vi "sort_points_iterative_closest_point.vi"(2 "Detected Camera Coordinates":cluster{"X":dbl, "Y":dbl}[](array[cluster]), 3 "Anticipated Camera Coordinates":cluster{"X":dbl, "Y":dbl}[](array[cluster]), 4 "Corresponding Projector Coordinates":cluster{"X":dbl, "Y":dbl}[](array[cluster])) -> (0 "Detected Camera Coordinates Sorted":cluster{"X":dbl, "Y":dbl}[](array[cluster]), 1 "Corresponding Projector Coordinates Filtered":cluster{"X":dbl, "Y":dbl}[](array[cluster]))   [LabVIEW 2019]
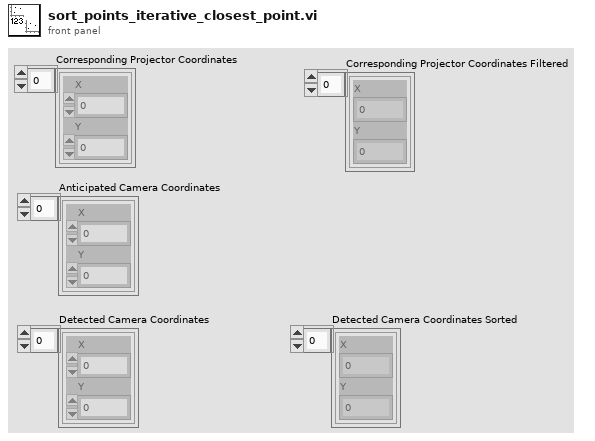
[diagram p1: front panel]
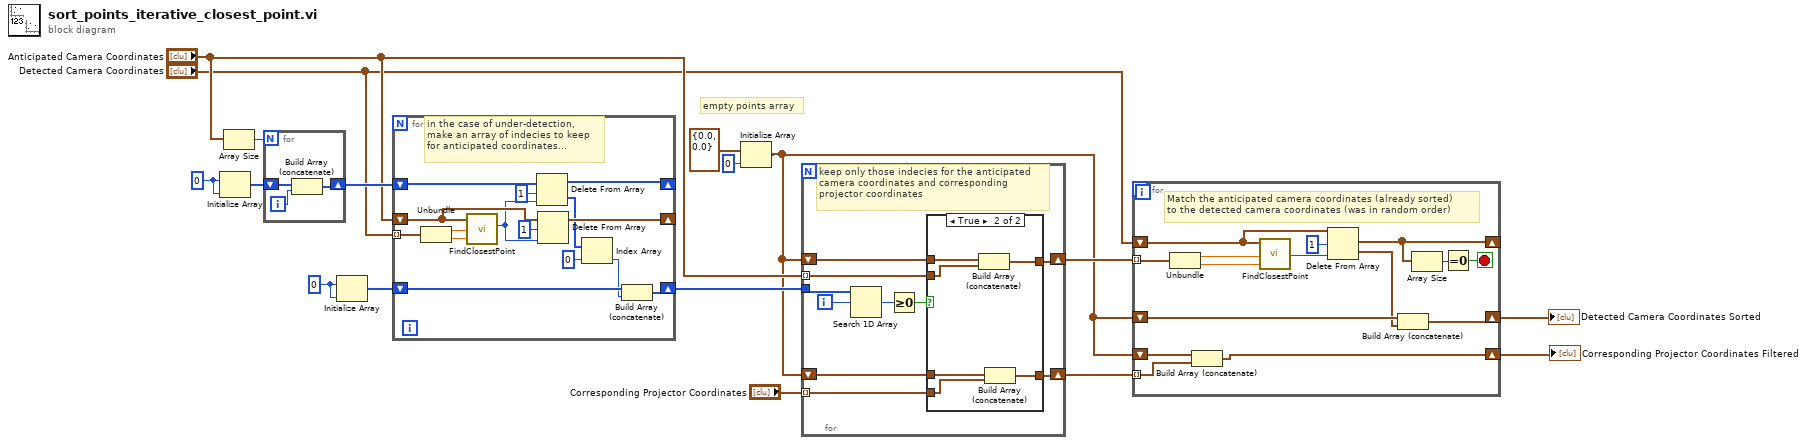
[diagram p0: block diagram]
diagram:
  w10 = 0
  w13 = 0
  # "empty points array"
  n1 = Initialize Array(w10, w10) -> (w8:i32[])
  n2 = Array Size(array="Anticipated Camera Coordinates") -> (size(s)=w9:i32)
  n3 = for {
    N: w9 -> [_]
    shift-right: [w20] -> w7
    shift-left: w8 -> [w19]
    i -> [w18]
    n4 = Build Array (concatenate)(w19, w18) -> (w20:i32[])
  }
  n5 = Initialize Array(w13, w13) -> (w14:i32[])
  n6 = for {
    tunnel: "Detected Camera Coordinates" -> [w35] mode=indexing
    shift-right: [w31] -> w15
    shift-left: w14 -> [w32]
    shift-right: [w29] -> _
    shift-left: "Anticipated Camera Coordinates" -> [w30]
    shift-right: [w26] -> _
    shift-left: w7 -> [w27]
    # "in the case of under-detection, \nmake an array of indecies to keep\nfor anticipated coordinates..."
    n7 = Unbundle(w35) -> ("X"=w34:dbl, "Y"=w33:dbl)
    n8 = call "FindClosestPoint.vi"("Y"=w33, "X"=w34, "Points"=w30) -> ("ShortestDistanceIndex"=w24:i32)  [unwired: 7 in, 1 out]
    n9 = Delete From Array(array=w27, length=1, index=w24) -> (deleted portion=w23:i32[], array with subset deleted=w26:i32[])
    n10 = Delete From Array(array=w30, length=1, index=w24) -> (array with subset deleted=w29:cluster{"X":dbl, "Y":dbl}[])  [unwired: 1 out]
    n11 = Index Array(array=w23, index=0) -> (element=w21:i32)
    n12 = Build Array (concatenate)(w32, w21) -> (w31:i32[])
  }
  n13 = Initialize Array(cluster{"X":dbl, "Y":dbl} {"X"=0.0, "Y"=0.0}, 0) -> (w2:cluster{"X":dbl, "Y":dbl}[])
  n14 = for {
    tunnel: "Anticipated Camera Coordinates" -> [w39] mode=indexing
    tunnel: w15 -> [w45]
    shift-right: [w41] -> w5
    shift-left: w2 -> [w40]
    shift-right: [w37] -> w1
    shift-left: w2 -> [w38]
    tunnel: "Corresponding Projector Coordinates" -> [w36] mode=indexing
    i -> [w44]
    # "keep only those indecies for the anticipated\ncamera coordinates and corresponding\nprojector coordinates"
    n15 = Search 1D Array(1D array=w45, element=w44) -> (index of element=w43:i32)  [unwired: 1 in]
    n16 = Greater Or Equal To 0?(x=w43) -> (x >= 0?=w42:bool)
    n17 = case shown="True" w42 {
      tunnel: [w47 w53] -> w41
      tunnel: w40 -> [w47 w52]
      tunnel: w39 -> [_ w51]
      tunnel: w38 -> [w46 w50]
      tunnel: [w46 w49] -> w37
      tunnel: w36 -> [_ w48]
      frame False {
      }
      frame True {
        n18 = Build Array (concatenate)(w52, w51) -> (w53:cluster{"X":dbl, "Y":dbl}[])
        n19 = Build Array (concatenate)(w50, w48) -> (w49:cluster{"X":dbl, "Y":dbl}[])
      }
    }
  }
  n20 = for {
    tunnel: w5 -> [w56] mode=indexing
    shift-right: [w62] -> w17
    shift-left: w2 -> [w63]
    shift-right: [w60] -> _
    shift-left: "Detected Camera Coordinates" -> [w66]
    shift-right: [w55] -> w16
    shift-left: w2 -> [w57]
    tunnel: w1 -> [w54] mode=indexing
    stop <- w58 stop-if-true
    # "Match the anticipated camera coordinates (already sorted) \nto the detected camera coordinates (was in random order)"
    n21 = Unbundle(w56) -> ("X"=w68:dbl, "Y"=w67:dbl)
    n22 = Build Array (concatenate)(w57, w54) -> (w55:cluster{"X":dbl, "Y":dbl}[])
    n23 = call "FindClosestPoint.vi"("Y"=w67, "X"=w68, "Points"=w66) -> ("ShortestDistanceIndex"=w64:i32)  [unwired: 7 in, 1 out]
    n24 = Delete From Array(array=w66, length=1, index=w64) -> (deleted portion=w61:cluster{"X":dbl, "Y":dbl}[], array with subset deleted=w60:cluster{"X":dbl, "Y":dbl}[])
    n25 = Build Array (concatenate)(w63, w61) -> (w62:cluster{"X":dbl, "Y":dbl}[])
    n26 = Array Size(array=w60) -> (size(s)=w59:i32)
    n27 = Equal To 0?(x=w59) -> (x = 0?=w58:bool)
  }
  "Detected Camera Coordinates Sorted" <- w17
  "Corresponding Projector Coordinates Filtered" <- w16
